vi "Write TTL.vi"(8 "error in (no error)":errorcluster, 10 "TTL":refnum<class "TTLController.lvclass">[](array[class]), 11 "Timeout in":refnum<class "Timeout.lvclass">) -> (0 "error out":errorcluster, 3 "Timeout out":refnum<class "Timeout.lvclass">)   [LabVIEW 2020, in "Timeout.lvclass"]
uses:
  Timeout.lvclass
  TTL VIs/Control Classes/Base Class/TTLController.lvclass
  Timeout.lvclass/Timeout.ctl
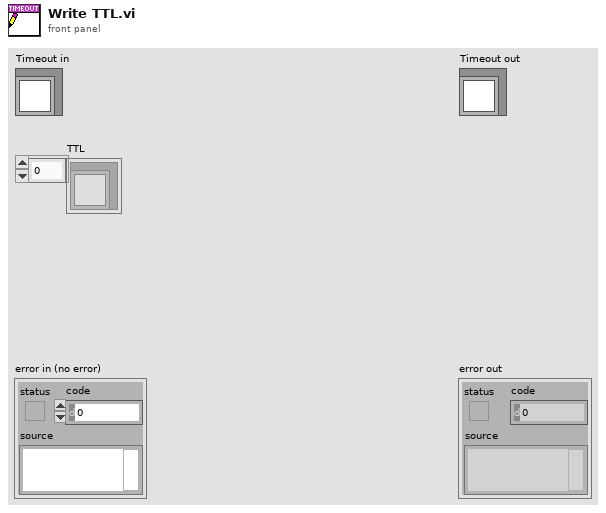
[diagram p1: front panel]
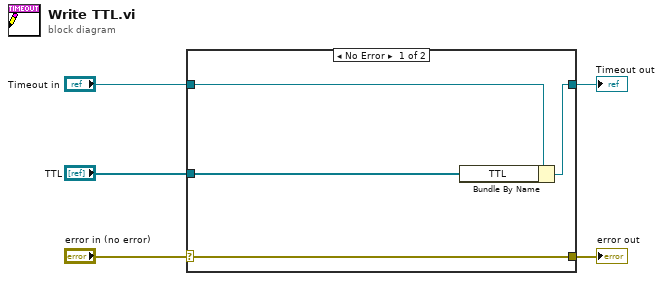
[diagram p0: block diagram]
diagram:
  n1 = case shown="No Error" "error in (no error)" {
    selector: "error in (no error)" -> [w9 w10]
    tunnel: [w9 w10] -> w4
    tunnel: [w7 w11] -> w2
    tunnel: "Timeout in" -> [w8 w11]
    tunnel: "TTL" -> [w6 _]
    frame No Error {
      n2 = Bundle By Name(cluster=w8, "TTL"=w6) -> (w7:refnum<class "Timeout.lvclass">)
    }
    frame Error {
    }
  }
  "error out" <- w4
  "Timeout out" <- w2
